vi "Send raw Gcode.vi"(8 "error in (no error)":errorcluster, 10 "Gcode":string, 11 "VISA resource name":refnum<visa-resource-name>) -> (0 "error out":errorcluster, 1 "command OK":bool, 2 "read buffer":string, 3 "VISA resource name out":refnum<visa-resource-name>)   [LabVIEW 2023, in "Marlin Instrument Driver.lvlib"]
doc: "Returns the current state of the configured X, Y, Z endstops. Takes into account any 'inverted endstop' settings, so one can confirm that the machine is interpreting the endstops correctly."
uses:
  Marlin Instrument Driver.lvlib
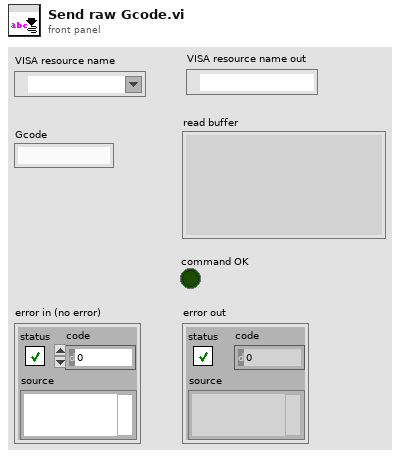
[diagram p1: front panel]
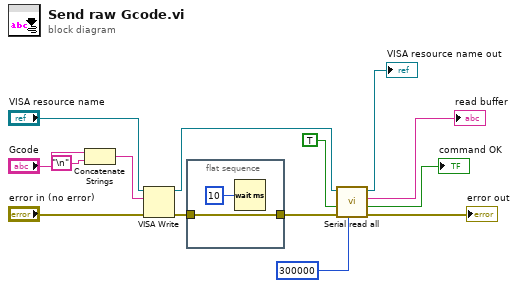
[diagram p0: block diagram]
diagram:
  n1 = Concatenate Strings("Gcode", "\n") -> (w12:string)
  n2 = VISA Write(VISA resource name="VISA resource name", write buffer=w12, error in (no error)="error in (no error)") -> (VISA resource name out=w11:refnum<visa-resource-name>, error out=w1:errorcluster)  [unwired: 1 out]
  n3 = flat-sequence {
    tunnel: [w15] -> w2
    tunnel: w1 -> [w15]
    frame #0 {
      n4 = Wait (ms)(milliseconds to wait=u32 10) -> ()  [unwired: 1 out]
    }
  }
  n5 = call "Serial read all.vi"("timeout (10000ms)"=u32 300000, "error in (no error)"=w2, "Wait for OK"=TRUE, "VISA Refnum in"=w11) -> ("error out"=→"error out":errorcluster, "command OK"=→"command OK":bool, "read buffer"=→"read buffer":string, "VISA Refnum out"=→"VISA resource name out":refnum<visa-resource-name>)  [unwired: 4 in]
